vi "Read Comm to Main.vi"(8 "error in (no error)":errorcluster, 11 "CIFTemplatePlugin in":refnum<class "Template_Plugin.lvclass">) -> (0 "error out":errorcluster, 3 "CIFTemplatePlugin out":refnum<class "Template_Plugin.lvclass">)   [LabVIEW 2021, in "Template_Plugin.lvclass"]
uses:
  Template_Plugin.lvclass
  Template_Plugin.lvclass/Template_Plugin.ctl
  525c214c-2a6b-4e7b-b3ce-0ad96b412d2f.vi
  Common/Typedef/OOB Comm/To Main Command.ctl
  Common/Template_Common.lvlib
  Common/Typedef/OOB Comm/To Main Command Data.ctl
  Common/Typedef/OOB Comm/To Main Command Payload.ctl
  4efb0375-f1de-4191-b03f-44d34e6646cb.vi
  <vilib>/CIF Foundation/CIF CIPC/TypeDefs/Read Position.ctl
  <vilib>/CIF Foundation/CIF CIPC/CIF_NI_CIPC.lvlib
  <vilib>/CIF Foundation/CIF CIPC/TypeDefs/Read Configuration.ctl
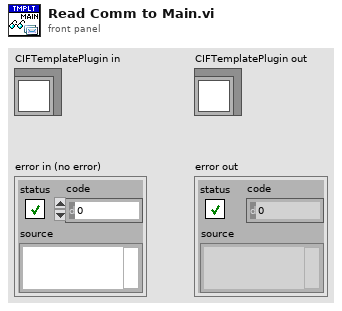
[diagram p1: front panel]
types:
  T1 = typedef "CIF_NI_CIPC.lvlib/Read Configuration.ctl" = cluster{"Read Position":T2, "Element Offset":i32, "Prepend Array Size":bool, "Get Read Position":bool}
  T2 = typedef "CIF_NI_CIPC.lvlib/Read Position.ctl" = enum16{"Next", "Newest", "Oldest", "Next Available", "Absolute"}
  T3 = typedef "Template_Common.lvlib/To Main Command Payload.ctl" = cluster{"Command":T4, "-> Main":T5}
  T4 = typedef "Template_Common.lvlib/To Main Command.ctl" = enum16{"Read Data", "Read DVR Data"}
  T5 = typedef "Template_Common.lvlib/To Main Command Data.ctl" = cluster{"Cmd Data 1 -> Main":i32}
  T6 = typedef "Template_Common.lvlib/To Main DVR Data.ctl" = cluster{"Data 1 DVR  -> Main":i32}
  T7 = typedef "Template_Common.lvlib/To Main Cyclic Data.ctl" = cluster{"Data 1 -> Main":i32}
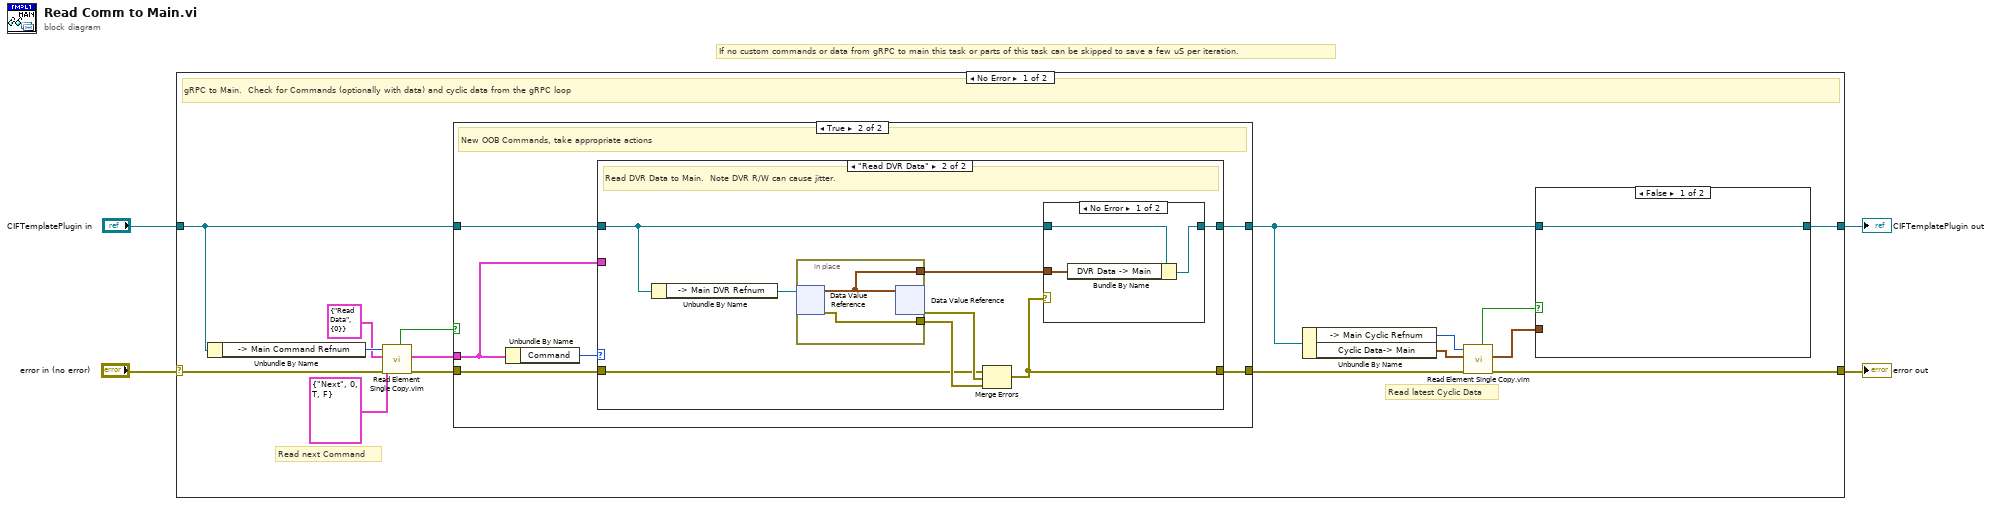
[diagram p0: block diagram]
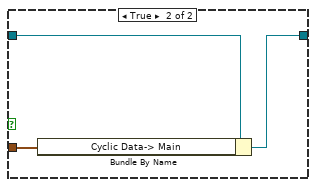
[diagram p2: hidden frame]
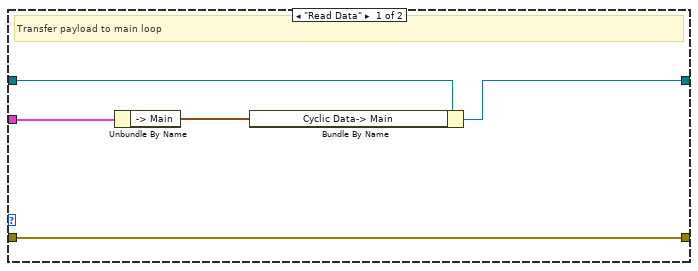
[diagram p4: hidden frame]
diagram:
  # "If no custom commands or data from gRPC to main this task or parts of this task can be skipped to save a few uS per iteration."
  n1 = case shown="No Error" "error in (no error)" {
    selector: "error in (no error)" -> [w19 w53]
    tunnel: [w11 w53] -> w3
    tunnel: [w5 w52] -> w1
    tunnel: "CIFTemplatePlugin in" -> [w18 w52]
    frame No Error {
      # "Read next Command"
      # "Read latest Cyclic Data"
      # "gRPC to Main.  Check for Commands (optionally with data) and cyclic data from the gRPC loop"
      n2 = Unbundle By Name(w18) -> ("-> Main Command Refnum"=w20:u64)
      n3 = call "Read Element Single Copy.vim"("error in (no error)"=w19, "Read Configuration"=T1 {"Read Position"=enum."Next", "Element Offset"=0, "Prepend Array Size"=TRUE, "Get Read Position"=FALSE}, "Data in"=T3 {"Command"=enum."Read Data", "-> Main"={"Cmd Data 1 -> Main"=0}} ("Payload"), "CIPC Reference in"=w20) -> ("error out"=w15:errorcluster, "Data out"=w14:T3, "Success"=w17:bool)  [unwired: 3 in, 2 out]
      n4 = case shown="True" w17 {
        tunnel: w18 -> [w26 w32]
        tunnel: [w26 w27] -> w6
        tunnel: w15 -> [w25 w31]
        tunnel: [w25 w30] -> w12
        tunnel: w14 -> [_ w28]
        frame False {
          # "No new OOB Commands"
        }
        frame True {
          # "New OOB Commands, take appropriate actions"
          n5 = Unbundle By Name(w28) -> ("Command"=w29:T4)
          n6 = case shown="\"Read DVR Data\"" w29 {
            tunnel: w31 -> [w37 w41]
            tunnel: w32 -> [w35 w40]
            tunnel: [w37 w38] -> w30
            tunnel: w28 -> [w36 _]
            tunnel: [w33 w39] -> w27
            frame "Read Data" {
              # "Transfer payload to main loop"
              n7 = Unbundle By Name(w36) -> ("-> Main"=w34:T5)
              n8 = Bundle By Name(cluster=w35, "Cyclic Data-> Main"=w34) -> (w33:refnum<class "Template_Plugin.lvclass">)
            }
            frame "Read DVR Data" {
              # "Read DVR Data to Main.  Note DVR R/W can cause jitter."
              n9 = Unbundle By Name(w40) -> ("-> Main DVR Refnum"=w43:refnum<data-value>)
              n10 = in-place {
                in-place-border: [w51] -> w45
                in-place-border: [w50] -> w42
                n11 = in-place-dvr #1(w43) -> (w50:T6, w51:errorcluster)
                n12 = in-place-dvr #1(w50) -> (w44:errorcluster)  [unwired: 1 out]
              }
              n13 = Merge Errors(w41, w44, w45) -> (w38:errorcluster)
              n14 = case shown="No Error" w38 {
                tunnel: w42 -> [w48 _]
                tunnel: w40 -> [w47 w49]
                tunnel: [w46 w49] -> w39
                frame No Error {
                  n15 = Bundle By Name(cluster=w47, "DVR Data -> Main"=w48) -> (w46:refnum<class "Template_Plugin.lvclass">)
                }
                frame Error {
                }
              }
            }
          }
        }
      }
      n16 = Unbundle By Name(w6) -> ("-> Main Cyclic Refnum"=w13:u64, "Cyclic Data-> Main"=w10:T7)
      n17 = call "Read Element Single Copy.vim"("error in (no error)"=w12, "Data in"=w10, "CIPC Reference in"=w13) -> ("error out"=w11:errorcluster, "Data out"=w7:T7, "Success"=w8:bool)  [unwired: 4 in, 2 out]
      n18 = case shown="False" w8 {
        tunnel: w7 -> [_ w23]
        tunnel: w6 -> [w21 w24]
        tunnel: [w21 w22] -> w5
        frame False {
        }
        frame True {
          n19 = Bundle By Name(cluster=w24, "Cyclic Data-> Main"=w23) -> (w22:refnum<class "Template_Plugin.lvclass">)
        }
      }
    }
    frame Error {
    }
  }
  "error out" <- w3
  "CIFTemplatePlugin out" <- w1
